vi "Stepper Sequence Change Focus Cam.vi"() -> ()   [LabVIEW 2013]
doc: "Writes specified digital values to all 14 digital I/O pins. Each pin must first be configured as a digital output using the Arduino Set Digital Pin Mode VI."
uses:
  Hello Optotune Lens (30.06.2014)/Calibration.ctl
  <vilib>/LabVIEW Interface for Arduino/Type Defs/Board Type.ctl
  <vilib>/Instr/_visa.llb/VISA Configure Serial Port (Instr).vi
  <vilib>/LabVIEW Interface for Arduino/LabVIEW Interface for Arduino.lvlib
panel:
  out "x/y":dbl=290.0
  in  "Schrittweite Fokus":i32=1
  in  "Stop (F)":bool
  out "Image 3":T1(plugin-control)
  in  "Anahl Messungen":i32=100
  out "Aktuelle Messung":i32
  in  "Maximaler Strom":dbl=290.0
  in  "Stepwidth X":dbl=4.0
  out "Aktueller Linsenstrom":dbl=289.0
  out "Schritt 7":bool
  out "Schritt 6":bool
  out "Schritt 5":bool
  out "Schritt 4":bool
  out "Schritt 3":bool
  out "Schritt 2":bool
  out "Schritt 1":bool=TRUE
  out "Value":u8
  out "x = y?":bool=TRUE
  in  "STOP INTIAL":bool
  out "VISA resource name out 3":refnum<visa-resource-name>="COM13"
  out "Command to Port 2":string
  out "Number of Measurements":i8=6
  in  "Min Focal Length 2":dbl
  in  "Max Focal Length":dbl=293.0
  out "Position_aktuell":dbl=19.0
  in  "First Motor Pin":u8=3
  in  "Pin Endlagenschalter":u8=32
  in  "Stepwidth Focalwidth lens":dbl=50.0
  in  "Calibration":T2={"Max Current A"=293.0, "Max Current B"=293.0, "UCL A"=300.0, "UCL B"=300.0, "LCL A"=0.0, "LCL B"=0.0} {"Max Current A" format="%#_g mA"; "Max Current B" format="%#_g mA"; "UCL A" format="%#_g mA"; "LCL A" format="%#_g mA"; "UCL B" format="%#_g mA"; "LCL B" format="%#_g mA"}
  out "ID":u16
  out "VISA resource name out":string="COM13"
  out "Calibration 2":T2={"Max Current A"=292.84, "Max Current B"=293.0, "UCL A"=292.76850585937495, "UCL B"=300.0, "LCL A"=4392.671494140624, "LCL B"=0.0} {"Max Current A" format="%#_g mA"; "Max Current B" format="%#_g mA"; "UCL A" format="%#_g mA"; "LCL A" format="%#_g mA"; "UCL B" format="%#_g mA"; "LCL B" format="%#_g mA"}
  out "OK":bool=TRUE
  out "Data":string
  out "Command to Port":string
  out "TA (°C)":dbl=38.5625
  out "error out":errorcluster={"status"=FALSE, "code"=1073676294, "source"="VISA Read in write read Lens Driver.vi->Stepper Sequence Change Focus Cam.vi"}
  in  "error in (no error)":errorcluster
  in  "VISA resource name":string="COM13"
  in  "Initial Speed":dbl
  # "Lens Settings"
  # "Measurement Settings"
  # "Initial Settings"
  # "mA"
  # "0 Fast, 100 slow"
  # "mA"
  # "Diodenstrom I0"
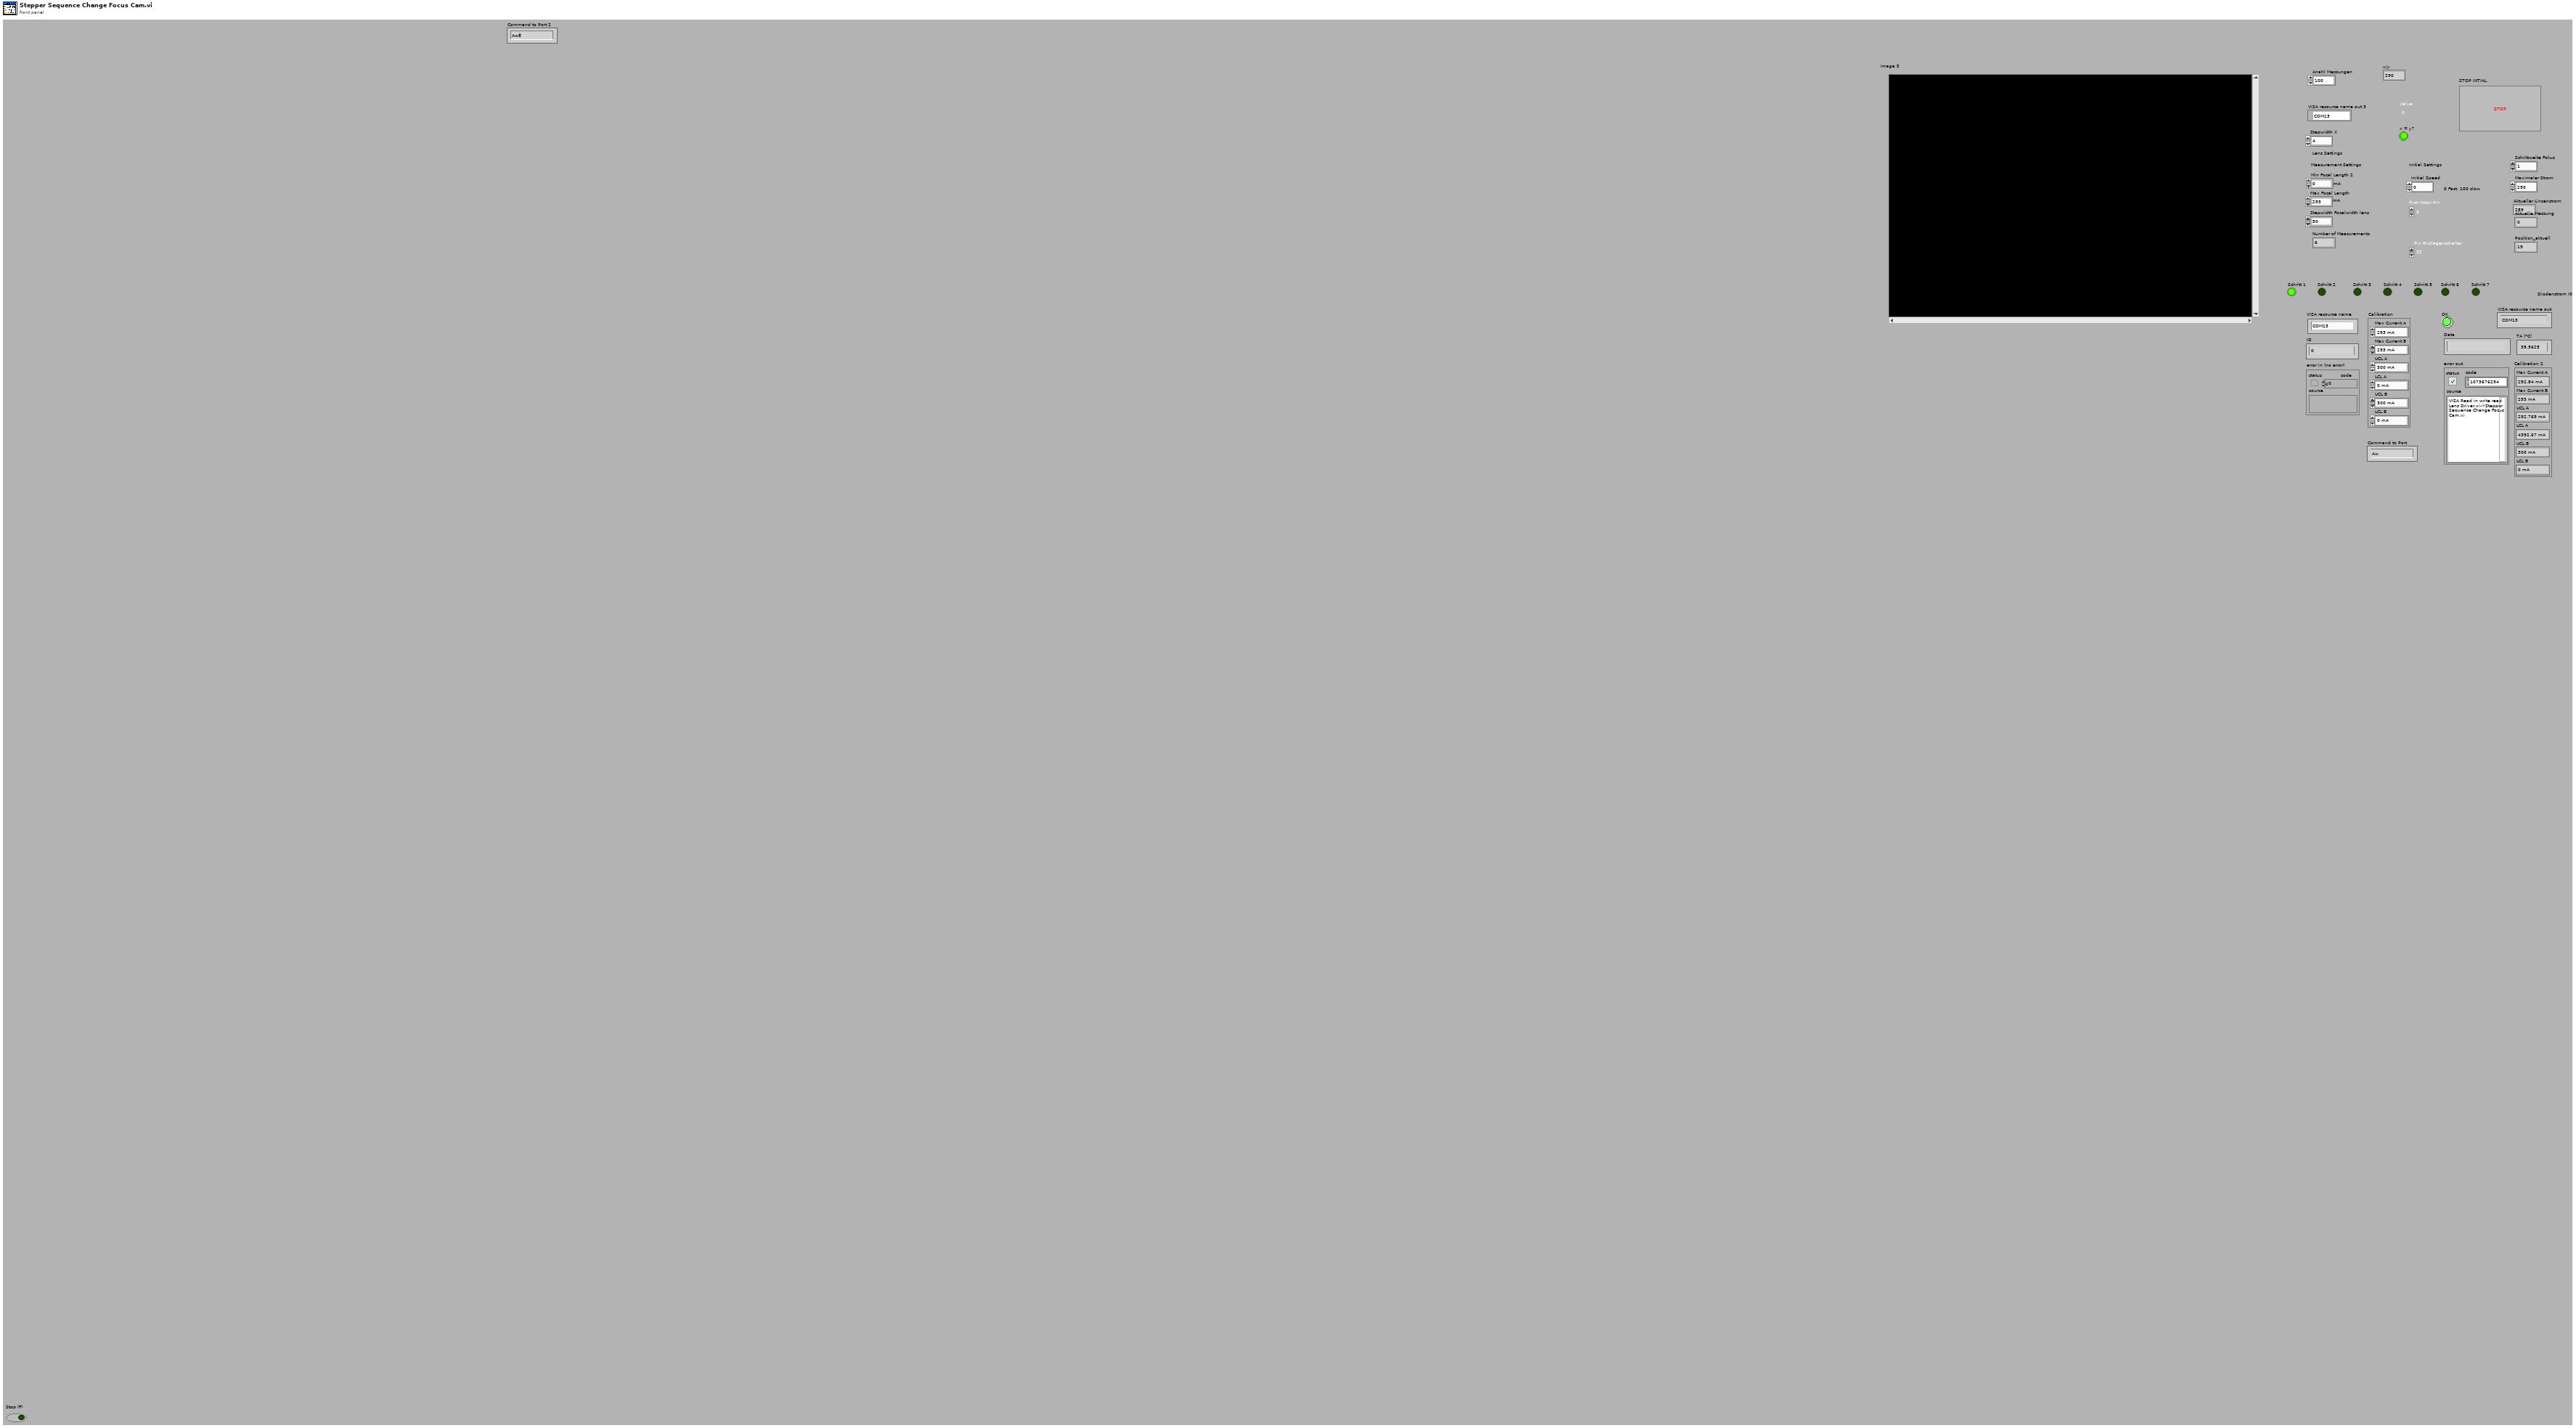
[diagram p1: front panel]
types:
  T1 = typedef "IMAQ Image.ctl" = refnum<image>
  T2 = typedef "Calibration.ctl" = cluster{"Max Current A":dbl, "Max Current B":dbl, "UCL A":dbl, "UCL B":dbl, "LCL A":dbl, "LCL B":dbl}
  T3 = typedef "LabVIEW Interface for Arduino.lvlib/Board Type.ctl" = enum16{"Uno", "Dimuelanove w/Atmega 328", "Mega 2560"}
  T4 = typedef "LabVIEW Interface for Arduino.lvlib/Arduino Resource.ctl" = cluster{"VISA resource":refnum<visa-resource-name>, "Board Type":T3, "Connection Type":enum8{"USB / Serial"}, "Bytes Per Packet (15)":u8}
diagram:
  n1 = flat-sequence {
    tunnel: [w43] -> w15
    tunnel: [w42] -> w14
    tunnel: [w41] -> w13
    tunnel: [w36] -> w5
    tunnel: [w35] -> w4
    tunnel: [w77] -> w25
    tunnel: [w76] -> w24
    tunnel: w15 -> [w99]
    tunnel: w14 -> [w98]
    tunnel: w13 -> [w97]
    tunnel: [w94] -> w12
    tunnel: [w78] -> w6
    tunnel: w5 -> [w77]
    tunnel: w4 -> [w76]
    tunnel: [w107] -> w19
    tunnel: w25 -> [w105]
    tunnel: [w106] -> w17
    tunnel: w24 -> [w108]
    tunnel: w12 -> [w104]
    tunnel: [w104] -> w11
    tunnel: [w103] -> w7
    tunnel: w6 -> [w103]
    tunnel: w19 -> [w129]
    tunnel: [w129] -> w18
    tunnel: w17 -> [w128]
    tunnel: [w128] -> w16
    tunnel: w11 -> [w127]
    tunnel: [w127] -> w10
    tunnel: [w126] -> w8
    tunnel: w7 -> [w126]
    tunnel: w18 -> [w133]
    tunnel: [w133] -> w23
    tunnel: w16 -> [w130]
    tunnel: [w130] -> w22
    tunnel: w10 -> [w132]
    tunnel: w8 -> [w131]
    tunnel: [w132] -> w3
    tunnel: [w131] -> w2
    tunnel: w23 -> [w144]
    tunnel: w22 -> [w143]
    tunnel: [w142] -> w21
    tunnel: [w141] -> w20
    tunnel: [w139] -> w9
    tunnel: w3 -> [w140]
    tunnel: w2 -> [w138]
    tunnel: [w136] -> w1
    tunnel: w21 -> [w283]
    tunnel: w20 -> [w282]
    tunnel: w9 -> [w279]
    tunnel: w1 -> [w280]
    frame #0 {
      w27 = FALSE ("Schritt 6")
      w63 = 2 ("length (rest)")
      w48 = u16 0 items=["None", "Last Bit", "TermChar", "Break"] ("Serial Settings:End Mode for Writes")
      w49 = u16 2 items=["None", "Last Bit", "TermChar"] ("Serial Settings:End Mode for Reads")
      # "Initialisierung des Arduinos"
      # "Initialisierung der Linse"
      # "Initialize Lens Driver"
      # "Initialize VISA port with correct parameters"
      n2 = local write "Schritt 6"(w27) -> ()
      n3 = local write "Schritt 5"(w27) -> ()
      n4 = local write "Schritt 4"(w27) -> ()
      n5 = local write "Schritt 3"(w27) -> ()
      n6 = local write "Schritt 2"(w27) -> ()
      n7 = local write "Schritt 7"(w27) -> ()
      n8 = Subtract(x="Max Focal Length", y="Min Focal Length 2") -> (x-y=w32:dbl)
      n9 = Divide(x=w32, y="Stepwidth Focalwidth lens") -> (x/y=w30:dbl)
      n10 = To Byte Integer(number=w30) -> (8bit integer=→"Number of Measurements":i8)
      n11 = call-poly "VISA Configure Serial Port"("VISA resource name"="VISA resource name", "timeout (10sec)"=u32 2000, "Enable Termination\nChar (T)"=FALSE ("Enable Termination\nChar (T)"), "baud rate (9600)"=u32 115200, "error in (no error)"="error in (no error)") -> ("VISA resource name out"=w53:refnum<visa-resource-name>, "error out"=w51:errorcluster)  [unwired: 9 in]
      n12 = property class="Instr"(reference=w53, error in=w51, "TermChar"=u8 10 ("Message Based Settings:Termination Character"), "ASRL End In"=w49, "ASRL End Out"=w48) -> (reference out=w52:refnum<visa-resource-name>, error out=w50:errorcluster)
      n13 = VISA Set I/O Buffer Size(VISA resource name=w52, error in (no error)=w50) -> (VISA resource name out=w45:refnum<visa-resource-name>, error out=w44:errorcluster)  [unwired: 2 in]
      n14 = VISA Flush I/O Buffer(VISA resource name=w45, error in (no error)=w44) -> (VISA resource name out=w65:refnum<visa-resource-name>)  [unwired: 1 in, 1 out]
      n15 = for {
        tunnel: w65 -> [w72]
        tunnel: [w69] -> w43
        tunnel: string[] ["Start", "MwDA", "CrMA00", "CrMB00", "CrUA00", "CrUB00", "CrLA00", "CrLB00", "PwTA\u0002Ð\u0001@"] -> [w67] mode=indexing
        tunnel: [w66] -> w59
        shift-right: [w70] -> w42
        shift-left: "Calibration" -> [w71]
        shift-right: [w68] -> w41
        shift-left: _ -> [w73]
        n16 = call "write read Lens Driver.vi"("VISA resource name"=w72, "command"=w67, "Calibration"=w71, "error in (no error)"=w73) -> ("VISA resource name out"=w69:refnum<visa-resource-name>, "Calibration 2"=w70:T2, "Data"=w66:string, "error out"=w68:errorcluster)  [unwired: 4 in, 4 out]
      }
      "VISA resource name out 3" <- w43
      n17 = String Subset(string=w59, offset (0)=w63, length (rest)=w63) -> (substring=w61:string)
      n18 = Type Cast(type=u16 0 ("length (rest)"), x=w61) -> (*(type *) &x=→"ID":u16)
      n19 = call <vilib>:"Init.vi"("VISA resource"=refnum<visa-resource-name> refnum, "Baud Rate (115200)"=u32 115200, "Board Type (Uno)"=Board_Type."Mega 2560") -> ("Arduino Resource"=w39:T4, "error out"=w40:errorcluster)  [unwired: 15 in]
      n20 = call <vilib>:"BlinkM Init.vi"("Arduino Resource"=w39, "error in"=w40) -> ("Arduino Resource"=w36:T4, "error out"=w35:errorcluster)  [unwired: 12 in]
      "Schritt 1" <- TRUE
    }
    frame #1 {
      # "Minimum Current"
      # "SET MIN Focus I=0"
      n21 = Unbundle By Name(w98) -> ("Max Current A"=w83:dbl)
      n22 = Divide(x=0.0, y=w83) -> (x/y=w90:dbl)
      n23 = Multiply(x=4096.0, y=w90) -> (x*y=w88:dbl)
      n24 = To Word Integer(number=w88) -> (16bit integer=w87:i16)
      n25 = Type Cast(x=w87) -> (*(type *) &x=w86:string)  [unwired: 1 in]
      n26 = Concatenate Strings("Aw", w86) -> (w84:string)
      "Command to Port" <- w84
      n27 = call "write read Lens Driver.vi"("VISA resource name"=w99, "command"=w84, "Calibration"=w98, "error in (no error)"=w97) -> ("VISA resource name out"=w96:refnum<visa-resource-name>, "Calibration 2"=→"Calibration 2":T2, "OK"=→"OK":bool, "Data"=→"Data":string, "error out"=w95:errorcluster)  [unwired: 4 in, 3 out]
      "VISA resource name out" <- w96
      n28 = call "write read Lens Driver.vi"("VISA resource name"=w96, "command"="TA", "error in (no error)"=w95) -> ("VISA resource name out"=w94:refnum<visa-resource-name>, "TA"=w80:u16, "error out"=w78:errorcluster)  [unwired: 5 in, 5 out]
      n29 = Multiply(x=w80, y=0.0625) -> (x*y=→"TA (°C)":dbl)
      "Schritt 2" <- TRUE
    }
    frame #2 {
      # "???? Richtige Richtung?"
      # "Move Right (Back to Origin)"
      # "Fahren, mit Initalgeschwindigkeit bis Endlage erreicht"
      n30 = local read "Initial Speed"() -> (w102:dbl)
      n31 = while {
        tunnel: w105 -> [w122]
        tunnel: w108 -> [w121]
        tunnel: TRUE -> [w119]
        tunnel: w102 -> [w120]
        tunnel: [w114] -> w107
        tunnel: [w113] -> w106
        stop <- w116 stop-if-true
        # "2"
        n32 = local read "First Motor Pin"() -> (w118:u8)
        n33 = call "Stepper_Sub_New.vi"("First Motor Pin"=w118, "error in"=w121, "Direction"=w119, "Velocity"=w120, "Arduino Resource"=w122) -> ("error out"=w111:errorcluster, "Arduino Resource 2"=w110:T4)  [unwired: 5 in]
        n34 = call <vilib>:"Digital Read Pin.vi"("Arduino Resource"=w110, "Digital I/O Pin (0)"="Pin Endlagenschalter", "error in"=w111) -> ("Arduino Resource"=w114:T4, "Value"=w112:u8, "error out"=w113:errorcluster)  [unwired: 10 in]
        "Value" <- w112
        n35 = Equal?(x=u8 0, y=w112) -> (x = y?=w117:bool)
        "x = y?" <- w117
        n36 = Or(x=w117, y="STOP INTIAL") -> (x .or. y?=w116:bool)
      }
      "Schritt 3" <- TRUE
    }
    frame #3 {
      # "???? RICHTIGE RICHTUNG?"
      # "Move to other direction"
      # "First Direction: Left"
      # "Position Zero"
      n37 = local write "Position_aktuell"(0.0 ("Position_aktuell")) -> ()
      "Schritt 4" <- TRUE
    }
    frame #4 {
      "Schritt 5" <- TRUE
    }
    frame #5 {
      n38 = for {
        N: "Anahl Messungen" -> [_]
        tunnel: w144 -> [w158]
        tunnel: w143 -> [w157]
        tunnel: [w156] -> w142
        tunnel: [w155] -> w141
        tunnel: w140 -> [w153]
        tunnel: w138 -> [w152]
        tunnel: [w150] -> w139
        tunnel: [w146] -> w136
        i -> [w151]
        n39 = flat-sequence {
          tunnel: w158 -> [w168]
          tunnel: w157 -> [w166]
          tunnel: [w167] -> w154
          tunnel: w153 -> [w172]
          tunnel: w152 -> [w169]
          tunnel: w151 -> [w163]
          tunnel: [w171] -> w150
          tunnel: [w170] -> _
          tunnel: [w165] -> w147
          tunnel: [w164] -> w146
          tunnel: [w163] -> w145
          tunnel: [w161] -> _
          tunnel: w154 -> [w238]
          tunnel: [w237] -> w149
          tunnel: [w236] -> w148
          tunnel: w147 -> [w235]
          tunnel: w145 -> [w234]
          tunnel: [w277] -> w155
          tunnel: [w278] -> w156
          tunnel: w149 -> [w278]
          tunnel: w148 -> [w277]
          frame #0 {
            n40 = Divide(x="Maximaler Strom", y="Schrittweite Fokus") -> (x/y=w159:dbl)
            "x/y" <- w159
            n41 = for {
              N: w159 -> [_]
              tunnel: w172 -> [w184]
              tunnel: [w183] -> w171
              tunnel: [w182] -> w170 mode=indexing
              tunnel: w169 -> [w181]
              tunnel: w168 -> [w180]
              tunnel: [w179] -> w167
              tunnel: w166 -> [w178]
              tunnel: [w177] -> w165
              tunnel: [w176] -> w164
              tunnel: [w174] -> w161 mode=indexing
              tunnel: "Schrittweite Fokus" -> [w173]
              i -> [w175]
              n42 = flat-sequence {
                tunnel: w184 -> [w195]
                tunnel: w181 -> [w194]
                tunnel: [w188] -> w182
                tunnel: [w192] -> w186
                tunnel: [w191] -> w185
                tunnel: w175 -> [w189]
                tunnel: w173 -> [w187]
                tunnel: [w223] -> w183
                tunnel: w186 -> [w224]
                tunnel: w185 -> [w223]
                tunnel: w180 -> [w221]
                tunnel: w178 -> [w220]
                tunnel: [w221] -> w177
                tunnel: [w220] -> w179
                tunnel: [w224] -> w176
                tunnel: [w222] -> w174
                frame #0 {
                  n43 = Multiply(x=w189, y=w187) -> (x*y=w188:i32)
                  "Aktueller Linsenstrom" <- w188
                  n44 = local read "Calibration"() -> (w190:T2)
                  n45 = Unbundle By Name(w190) -> ("Max Current A"=w193:dbl)
                  n46 = Divide(x=w188, y=w193) -> (x/y=w202:dbl)
                  n47 = Multiply(x=4096.0, y=w202) -> (x*y=w200:dbl)
                  n48 = To Word Integer(number=w200) -> (16bit integer=w199:i16)
                  n49 = Type Cast(x=w199) -> (*(type *) &x=w198:string)  [unwired: 1 in]
                  n50 = Concatenate Strings("Aw", w198) -> (w196:string)
                  "Command to Port 2" <- w196
                  n51 = call "write read Lens Driver.vi"("VISA resource name"=w195, "command"=w196, "Calibration"=w190, "error in (no error)"=w194) -> ("VISA resource name out"=w192:refnum<visa-resource-name>, "error out"=w191:errorcluster)  [unwired: 4 in, 6 out]
                }
                frame #1 {
                  # "Strip path so it gives\ncurrent VI directory"
                  # "Give current path of VI"
                  # "Read an image\nfrom file"
                  # "Get image type"
                  # "Image folder"
                  # "Create an image"
                  n52 = call "Vision Acquisition"("Stop (F)"="Stop (F)") -> ("Image Out"=w204:T1)  [unwired: 22 in, 4 out]
                  n53 = Wait (ms)(milliseconds to wait=u32 20) -> ()  [unwired: 1 out]
                  n54 = local read "Position_aktuell"() -> (w207:dbl)
                  n55 = local read "Aktueller Linsenstrom"() -> (w208:dbl)
                  n56 = Number To Decimal String(number=w207) -> (decimal integer string=w215:string)  [unwired: 1 in]
                  n57 = Strip Path(path=path "C:/Users/Bene/Dropbox/Dokumente/FHKoeln/Projekt Master/Labview/Bilder/Bild/Focus" ("base path")) -> (stripped path=w218:path)  [unwired: 1 out]
                  n58 = Search and Replace String(input string="step_j-fokus_i.png" ("name or relative path"), search string="j", replace string=w215) -> (result string=w212:string)  [unwired: 5 in, 3 out]
                  n59 = Number To Decimal String(number=w208) -> (decimal integer string=w211:string)  [unwired: 1 in]
                  n60 = Search and Replace String(input string=w212, search string="i", replace string=w211) -> (result string=w209:string)  [unwired: 5 in, 3 out]
                  n61 = Build Path(base path=w218, name or relative path=w209) -> (appended path=w214:path)
                  n62 = local read "Position_aktuell"() -> (w222:dbl)
                  n63 = call-poly "IMAQ Write File 2"("File Path"=w214, "Image"=w204) -> ("Image Out (duplicate)"=→"Image 3":T1)  [unwired: 8 in, 1 out]
                  n64 = Wait (ms)(milliseconds to wait=u32 20) -> ()  [unwired: 1 out]
                }
              }
            }
            "Aktuelle Messung" <- w163
          }
          frame #1 {
            n65 = flat-sequence {
              tunnel: w238 -> [w240]
              tunnel: [w240] -> w233
              tunnel: ["Stepwidth X"] -> w232
              tunnel: [w242] -> w231
              tunnel: [w241] -> w230
              tunnel: w235 -> [w241]
              tunnel: w234 -> [_]
              tunnel: [w256] -> w228
              tunnel: [w255] -> w229
              tunnel: w233 -> [w257]
              tunnel: w232 -> [w252]
              tunnel: w231 -> [w253]
              tunnel: w230 -> [w250]
              tunnel: [w248] -> w227
              tunnel: w229 -> [w273]
              tunnel: w228 -> [w274]
              tunnel: [w274] -> w226
              tunnel: [w273] -> w225
              tunnel: w227 -> [w272]
              tunnel: [w275] -> w236
              tunnel: [w276] -> w237
              tunnel: w226 -> [w276]
              tunnel: w225 -> [w275]
              frame #0 {
                # "???? RICHTIGE RICHTUNG?"
                n66 = Greater?(x="Stepwidth X", y=0.0) -> (0:w245:bool)
                n67 = Select(t=TRUE, s=w245, f=FALSE) -> (s? t:f=w242:bool)
              }
              frame #1 {
                n68 = local read "Position_aktuell"() -> (w249:dbl)
                n69 = local read "Initial Speed"() -> (w254:dbl)
                n70 = Absolute Value(x=w252) -> (abs(x)=w251:dbl)
                n71 = Increment(x=w251) -> (x+1=w247:dbl)
                n72 = for {
                  N: w247 -> [_]
                  tunnel: w257 -> [w266]
                  tunnel: [w269] -> w256
                  tunnel: [w268] -> w255
                  tunnel: w254 -> [w271]
                  tunnel: w253 -> [w265]
                  tunnel: w250 -> [w267]
                  tunnel: w249 -> [w259]
                  tunnel: [w258] -> w248
                  i -> [w261]
                  n73 = Select(t=1.0, s=w265, f=-1.0) -> (s? t:f=w262:dbl)
                  n74 = local read "First Motor Pin"() -> (w270:u8)
                  n75 = Multiply(x=w262, y=w261) -> (x*y=w260:dbl)
                  n76 = Add(x=w260, y=w259) -> (x+y=w258:dbl)
                  n77 = call "Stepper_Sub_New.vi"("First Motor Pin"=w270, "error in"=w266, "Direction"=w265, "Velocity"=w271, "Arduino Resource"=w267) -> ("error out"=w268:errorcluster, "Arduino Resource 2"=w269:T4)  [unwired: 5 in]
                }
              }
              frame #2 {
                n78 = local write "Position_aktuell"(w272) -> ()
              }
              frame #3 {
              }
            }
          }
          frame #2 {
          }
        }
      }
      "Schritt 6" <- TRUE
    }
    frame #6 {
      n79 = call <vilib>:"Close.vi"("Arduino Resource"=w283, "error in"=w282) -> ("error out"=w286:errorcluster)  [unwired: 13 in]
      n80 = VISA Close(VISA resource name=w280, error in (no error)=w279) -> (error out=w284:errorcluster)
      n81 = call <vilib>:"Simple Error Handler.vi"("error in (no error)"=w286) -> ()  [unwired: 4 in, 5 out]
      n82 = call <vilib>:"Simple Error Handler.vi"("error in (no error)"=w284) -> ("error out"=→"error out":errorcluster)  [unwired: 4 in, 4 out]
      "Schritt 7" <- TRUE
    }
  }
